vi "HostInteractiveOverlayedGraph.vi"(8 "stop_sign_queue":refnum<queue>, 11 "InputImg":i32[][](array[numeric])) -> (0 "Break":bool, 3 "Output_Coord":dbl[][](array[numeric]))   [LabVIEW 2024]
panel:
  in  "Revert":bool
  in  "stop":bool
  out "Image":i32[][](graph)
  out "Two Point Clicked?":bool
  in  "Ok":bool
  out "Point Clicked":i32
  in  "Reset":bool
  out "vidx":i32
  out "hidx":i32
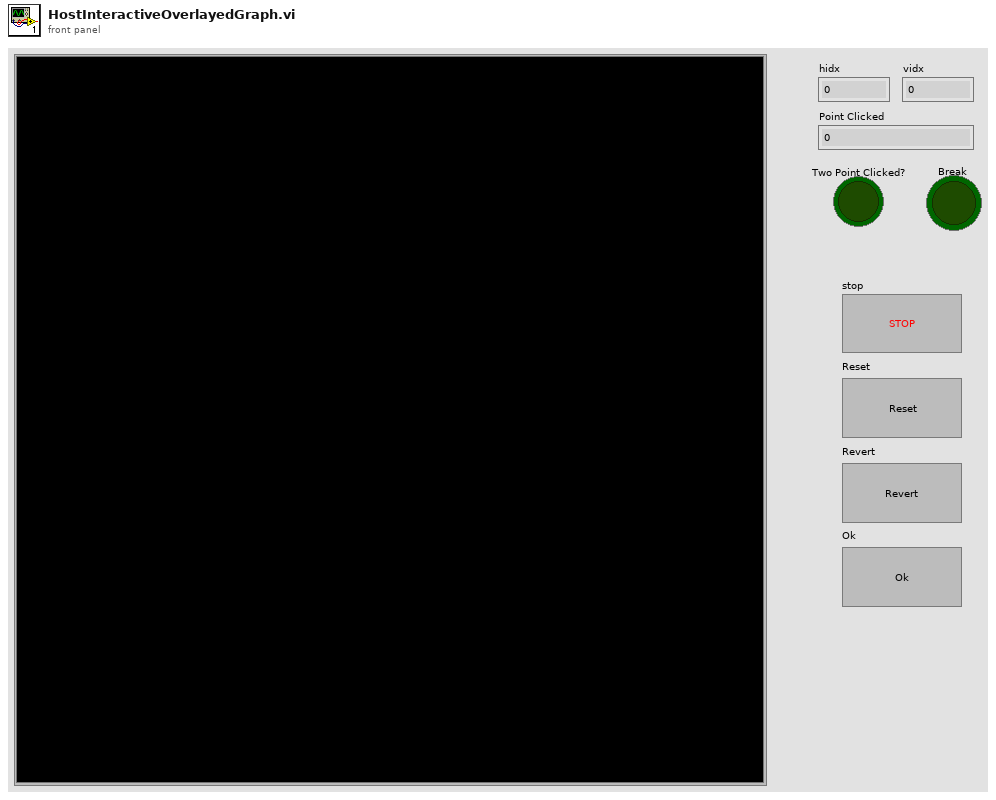
[diagram p1: front panel]
types:
  T1 = cluster{"Width":i16, "Style":enum32{"Solid", "Dash", "Dot", "DashDot", "DashDotDot"}}
  T2 = typedef "LVPoint32TypeDef.ctl" = cluster{"Horizontal":i32, "Vertical":i32}
  T3 = typedef "LVRectTypeDef.ctl" = cluster{"Left":i16, "Top":i16, "Right":i16, "Bottom":i16}
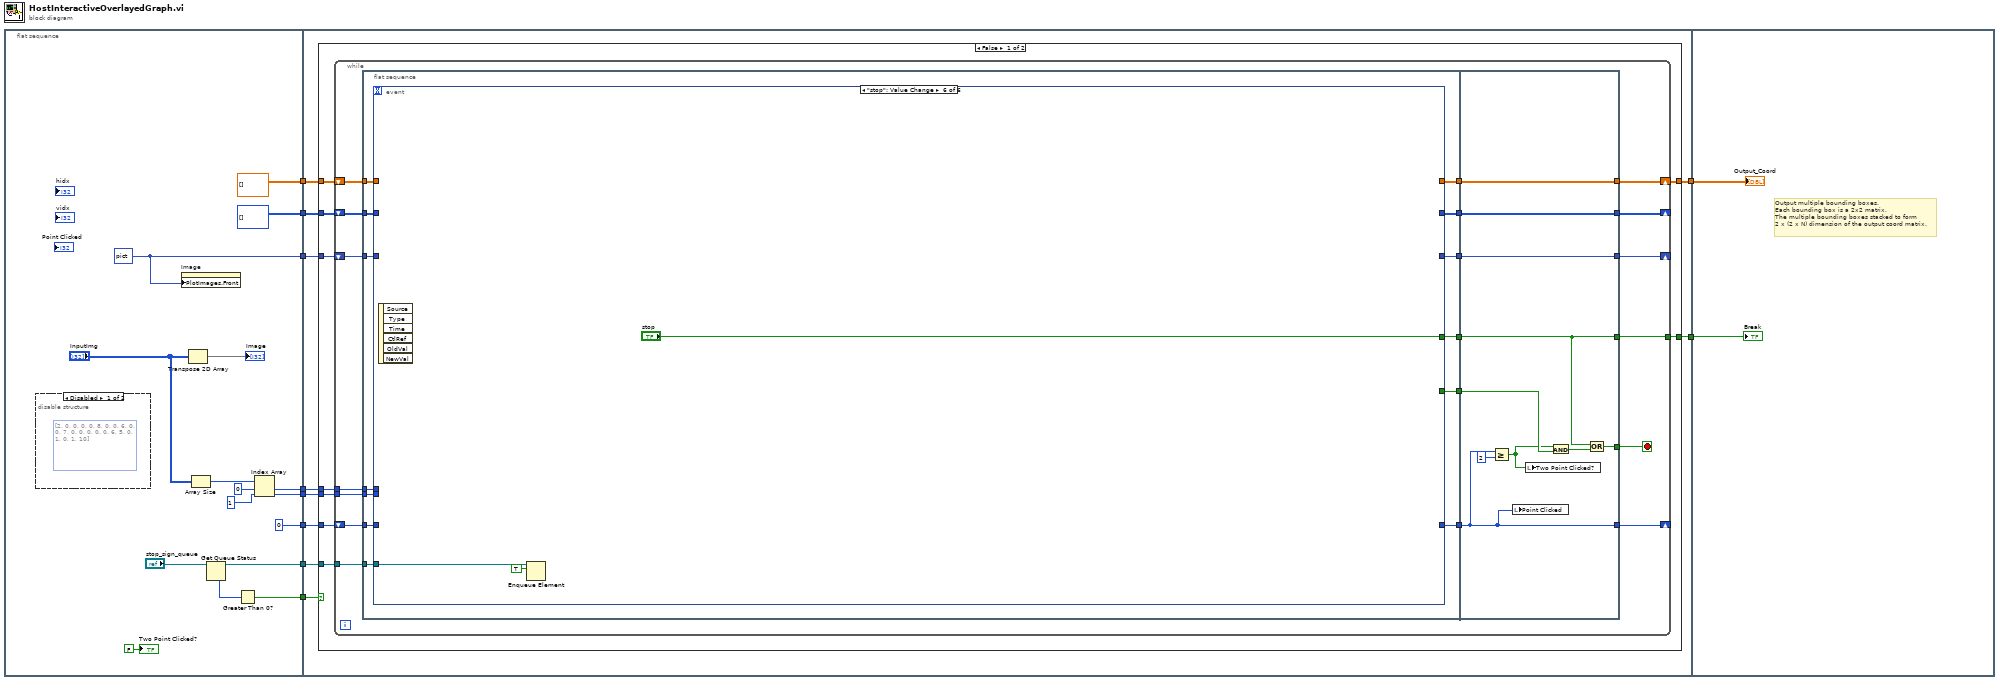
[diagram p0: block diagram]
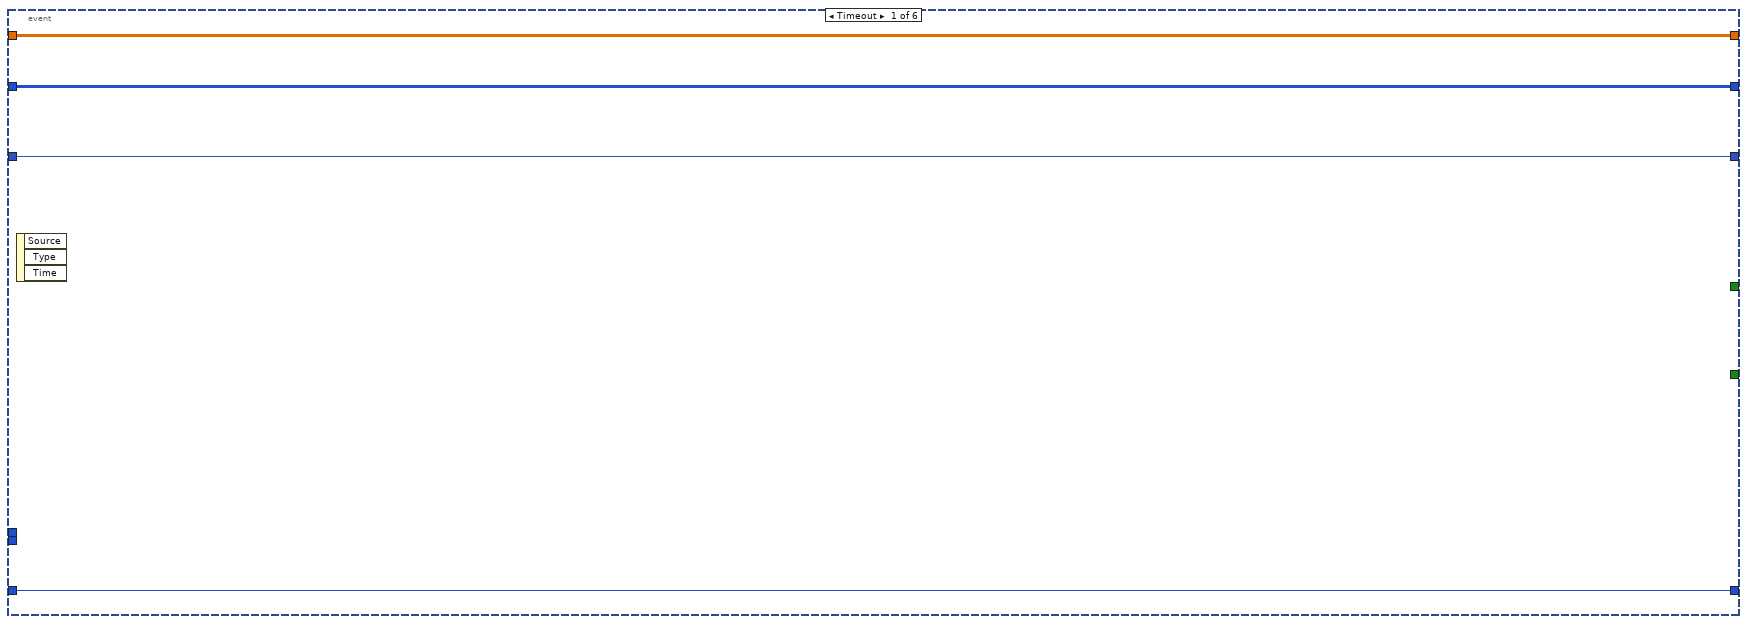
[diagram p3: hidden frame]
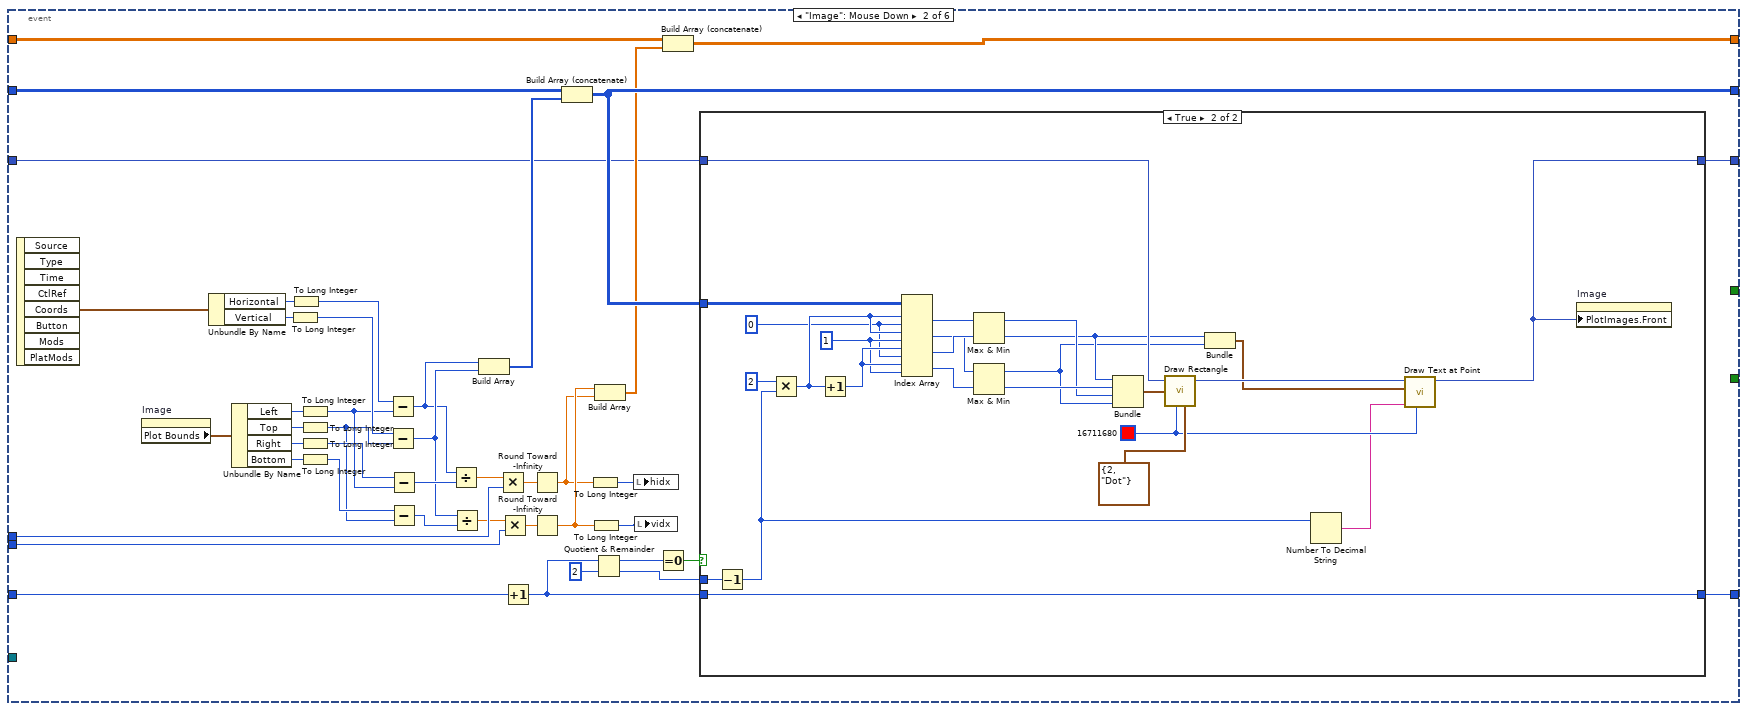
[diagram p4: hidden frame]
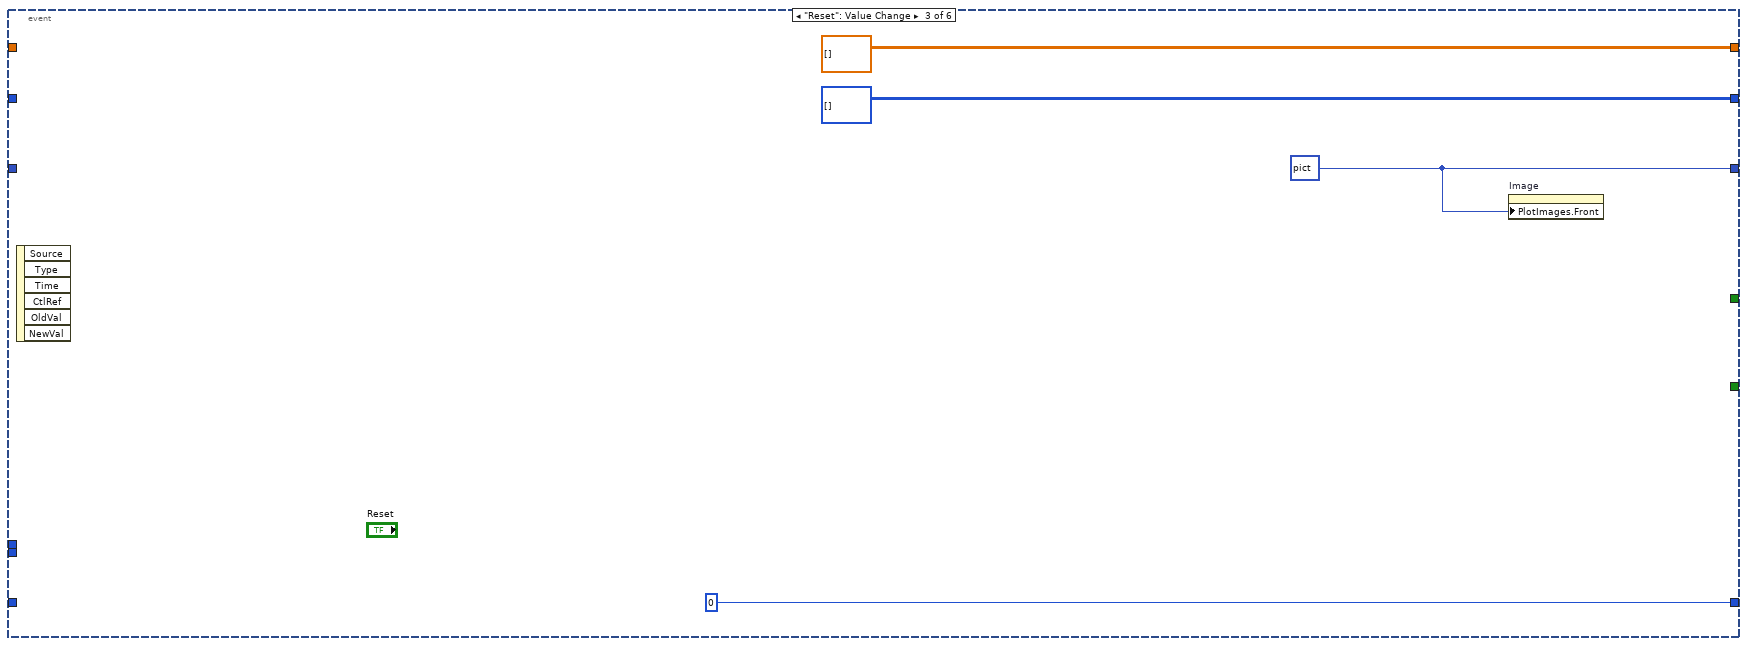
[diagram p6: hidden frame]
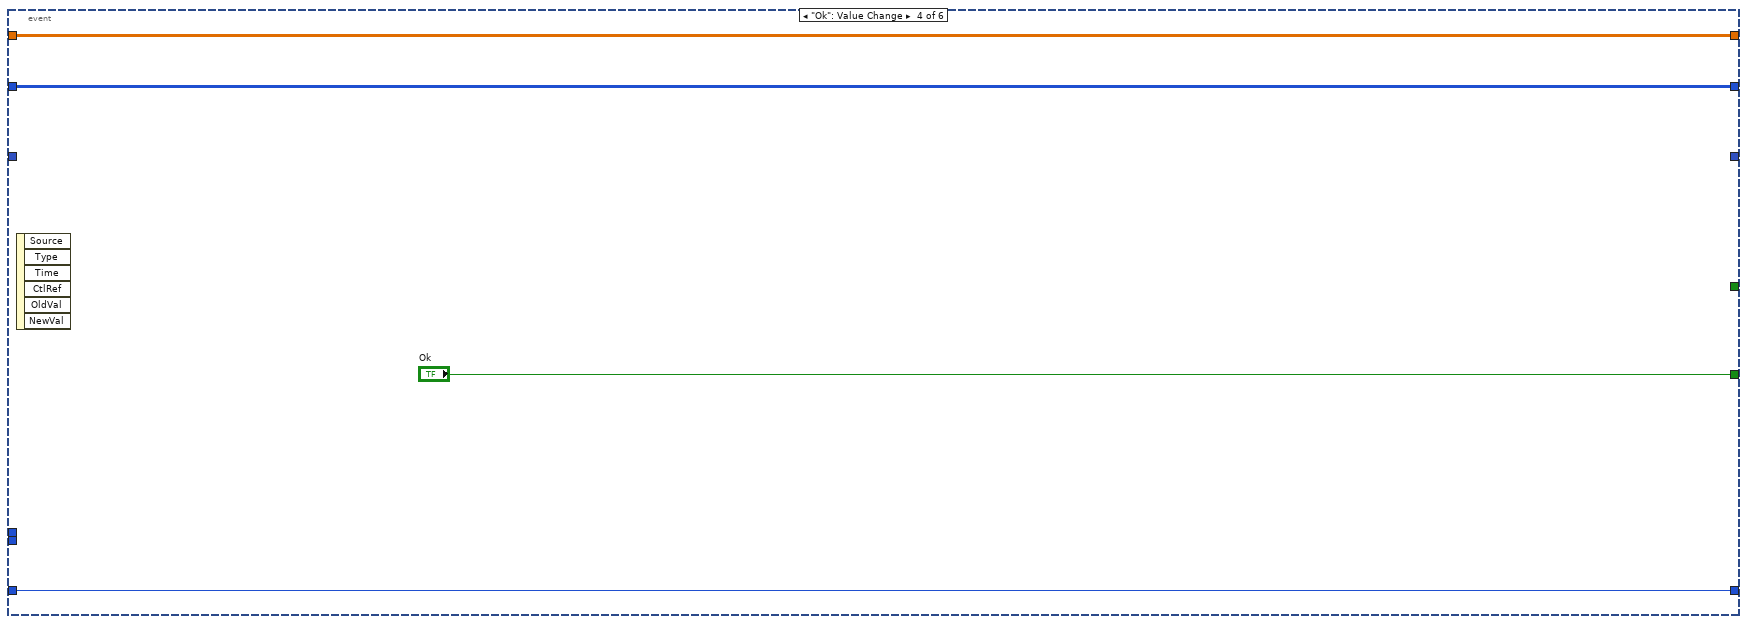
[diagram p7: hidden frame]
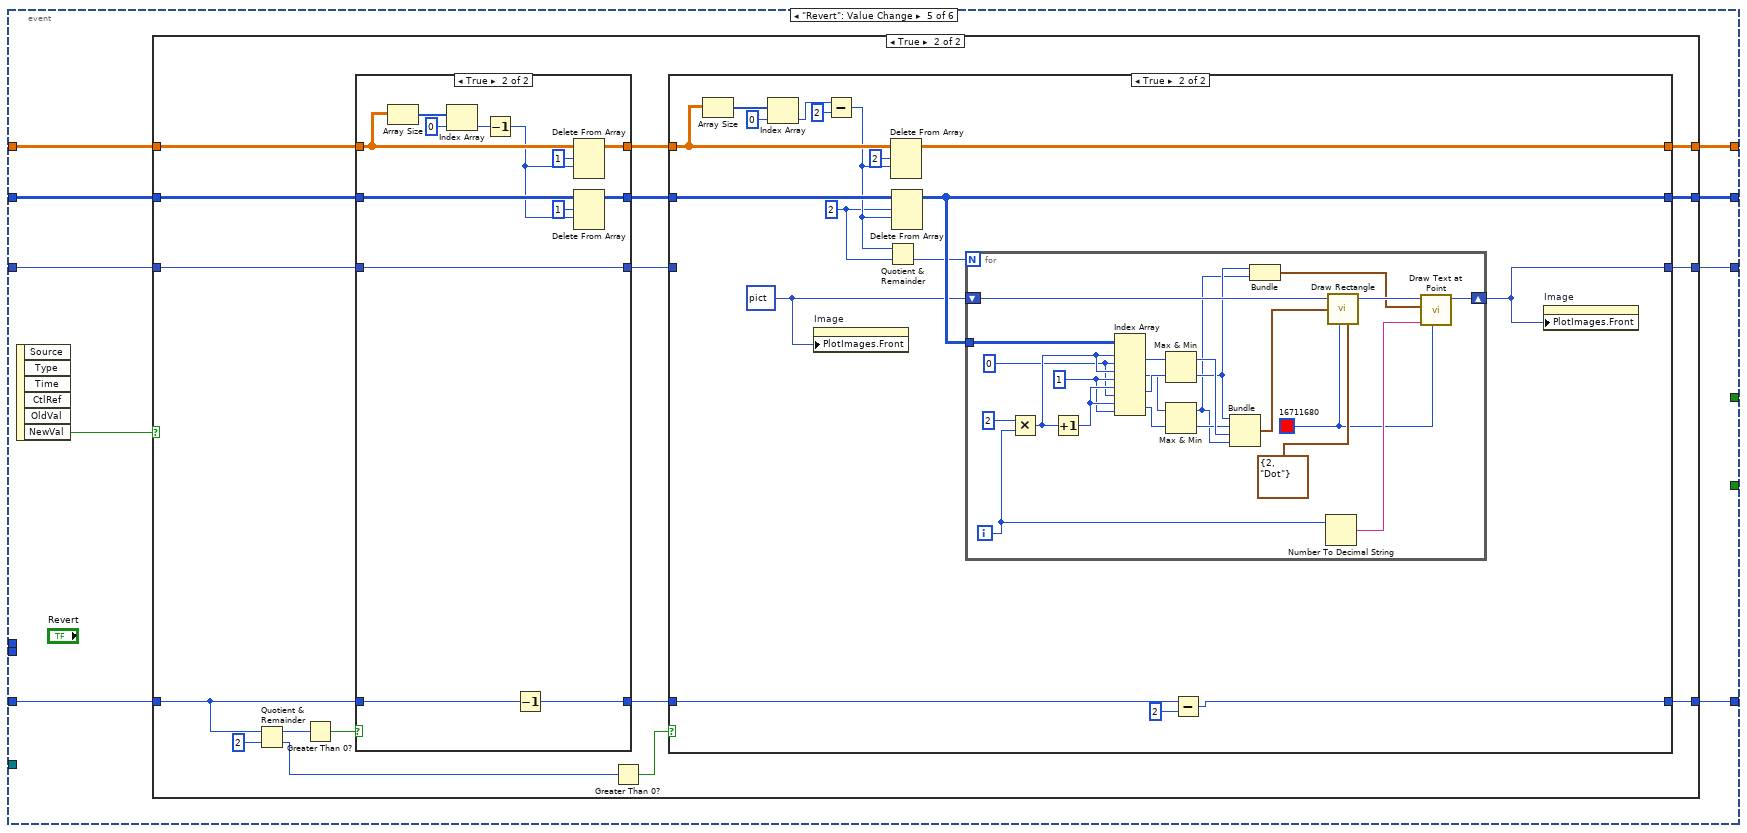
[diagram p8: hidden frame]
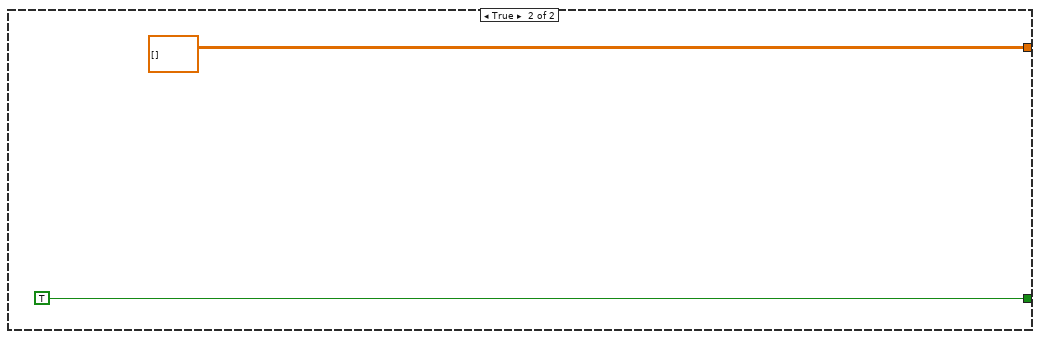
[diagram p12: hidden frame]
diagram:
  n1 = flat-sequence {
    tunnel: [w23] -> w10
    tunnel: [w22] -> w9
    tunnel: [0] -> w8
    tunnel: [dbl[][] []] -> w7
    tunnel: [w17] -> w4
    tunnel: [w16] -> w3
    tunnel: [i32[][] []] -> w2
    tunnel: [w14] -> w1
    tunnel: w10 -> [w36]
    tunnel: w9 -> [w35]
    tunnel: w8 -> [w34]
    tunnel: w7 -> [w33]
    tunnel: [w32] -> w6
    tunnel: [w31] -> w5
    tunnel: w4 -> [w30]
    tunnel: w3 -> [w29]
    tunnel: w2 -> [w28]
    tunnel: w1 -> [w27]
    tunnel: w6 -> [w267]
    tunnel: w5 -> [w266]
    frame #0 {
      w14 = picture data[5B] ("picture")
      n2 = disable-structure shown="Disabled" {
        frame Disabled {
          (unwired) i32[][] [[2, 0, 0, 0, 0, 8], [0, 0, 6, 0, 0, 7], [0, 0, 0, 0, 0, 6], [5, 0, 1, 0, 1, 10]]
        }
        frame Enabled {
        }
      }
      n3 = property on="Image" class="IntGraph (strict)"("PlotImages.Front"=w14) -> ()  [unwired: 2 in, 2 out]
      n4 = Transpose 2D Array(2D array="InputImg") -> (transposed array=→"Image":i32[][])
      n5 = Array Size(array="InputImg") -> (size(s)=w26:i32[])
      n6 = Get Queue Status(queue="stop_sign_queue") -> (queue out=w16:refnum<queue>, # elements in queue=w11:i32)  [unwired: 2 in, 6 out]
      n7 = Greater Than 0?(x=w11) -> (x > 0?=w17:bool)
      n8 = Index Array(array=w26, index #1=0 ("index"), index #2=1 ("index")) -> (element #1=w23:i32, element #2=w22:i32)
      "Two Point Clicked?" <- FALSE ("Two Point Clicked?")
    }
    frame #1 {
      n9 = case shown="False" w30 {
        tunnel: w36 -> [w45 _]
        tunnel: w35 -> [w44 _]
        tunnel: w34 -> [w43 _]
        tunnel: w33 -> [w42 _]
        tunnel: [w41 dbl[][] []] -> w32
        tunnel: [w40 TRUE ("stop")] -> w31
        tunnel: w29 -> [w39 _]
        tunnel: w28 -> [w38 _]
        tunnel: w27 -> [w37 _]
        frame False {
          n10 = while {
            tunnel: w45 -> [w64]
            tunnel: w44 -> [w63]
            shift-right: [w60] -> _
            shift-left: w43 -> [w62]
            shift-right: [w57] -> w41
            shift-left: w42 -> [w59]
            tunnel: [w53] -> w40
            tunnel: w39 -> [w52]
            shift-right: [w49] -> _
            shift-left: w38 -> [w51]
            shift-right: [w46] -> _
            shift-left: w37 -> [w48]
            stop <- w56 stop-if-true
            n11 = flat-sequence {
              tunnel: w64 -> [w77]
              tunnel: w63 -> [w76]
              tunnel: w62 -> [w75]
              tunnel: [w74] -> w61
              tunnel: w59 -> [w73]
              tunnel: [w72] -> w58
              tunnel: [w71] -> w55
              tunnel: [w70] -> w54
              tunnel: w52 -> [w69]
              tunnel: w51 -> [w68]
              tunnel: [w67] -> w50
              tunnel: w48 -> [w66]
              tunnel: [w65] -> w47
              tunnel: w61 -> [w254]
              tunnel: [w254] -> w60
              tunnel: w58 -> [w262]
              tunnel: [w262] -> w57
              tunnel: [w257] -> w56
              tunnel: w55 -> [w261]
              tunnel: w54 -> [w258]
              tunnel: [w258] -> w53
              tunnel: w50 -> [w256]
              tunnel: [w256] -> w49
              tunnel: w47 -> [w255]
              tunnel: [w255] -> w46
              frame #0 {
                n12 = event shown="[5] \"stop\": Value Change" {
                  selector: _ -> [_ _ _ _ _ _]
                  dyn-events: _ -> [_ _ _ _ _ _]
                  timeout: _ -> [_ _ _ _ _ _]
                  tunnel: w77 -> [_ w123 _ _ _ _]
                  tunnel: w76 -> [_ w122 _ _ _ _]
                  tunnel: w75 -> [w81 w119 _ w158 w168 _]
                  tunnel: [w81 w121 0 w158 w161 _] -> w74
                  tunnel: w73 -> [w80 w120 _ w159 w167 _]
                  tunnel: [w80 w118 dbl[][] [] w159 w164 _] -> w72
                  tunnel: [_ _ _ "Ok" _ _] -> w71
                  tunnel: [_ _ _ _ _ "stop"] -> w70
                  tunnel: w69 -> [_ _ _ _ _ w252]
                  tunnel: w68 -> [w79 w117 _ w156 w166 _]
                  tunnel: [w79 w116 i32[][] [] w156 w163 _] -> w67
                  tunnel: w66 -> [w78 w85 _ _ w165 _]
                  tunnel: [w78 w84 w152 _ w162 _] -> w65
                  event Timeout {
                    n13 = event-data() -> ()  [unwired: 1 in, 3 out]
                  }
                  event "Image": Mouse Down {
                    n14 = event-data() -> ("Coords"=w124:T2)  [unwired: 1 in, 7 out]
                    n15 = property on="Image" class="IntGraph (strict)"() -> ("Plot Bounds"=w96:T3)  [unwired: 2 in, 2 out]
                    n16 = Unbundle By Name(w124) -> ("Horizontal"=w115:i32, "Vertical"=w113:i32)
                    n17 = Unbundle By Name(w96) -> ("Left"=w111:i16, "Top"=w110:i16, "Right"=w109:i16, "Bottom"=w108:i16)
                    n18 = To Long Integer(number=w113) -> (32bit integer=w112:i32)
                    n19 = To Long Integer(number=w115) -> (32bit integer=w114:i32)
                    n20 = To Long Integer(number=w111) -> (32bit integer=w107:i32)
                    n21 = To Long Integer(number=w110) -> (32bit integer=w100:i32)
                    n22 = To Long Integer(number=w109) -> (32bit integer=w105:i32)
                    n23 = To Long Integer(number=w108) -> (32bit integer=w106:i32)
                    n24 = Subtract(x=w114, y=w107) -> (x-y=w86:i32)
                    n25 = Subtract(x=w112, y=w100) -> (x-y=w92:i32)
                    n26 = Subtract(x=w105, y=w107) -> (x-y=w104:i32)
                    n27 = Subtract(x=w106, y=w100) -> (x-y=w101:i32)
                    n28 = Divide(x=w86, y=w104) -> (x/y=w103:dbl)
                    n29 = Divide(x=w92, y=w101) -> (x/y=w102:dbl)
                    n30 = Build Array(w86, w92) -> (w93:i32[])
                    n31 = Multiply(x=w103, y=w123) -> (x*y=w99:dbl)
                    n32 = Multiply(x=w102, y=w122) -> (x*y=w98:dbl)
                    n33 = Increment(x=w119) -> (x+1=w88:i32)
                    n34 = Round Toward -Infinity(1:w99) -> (0:w94:dbl)
                    n35 = Round Toward -Infinity(1:w98) -> (0:w95:dbl)
                    n36 = Build Array (concatenate)(w117, w93) -> (w116:i32[][])
                    n37 = To Long Integer(number=w94) -> (32bit integer=w83:i32)
                    n38 = To Long Integer(number=w95) -> (32bit integer=w82:i32)
                    n39 = Quotient & Remainder(x=w88, y=2) -> (x-y*floor(x/y)=w90:i32, floor(x/y)=w87:i32)
                    n40 = Build Array(w95, w94) -> (w97:dbl[])
                    n41 = local write "hidx"(w83) -> ()
                    n42 = local write "vidx"(w82) -> ()
                    n43 = Equal To 0?(x=w90) -> (x = 0?=w89:bool)
                    n44 = Build Array (concatenate)(w120, w97) -> (w118:dbl[][])
                    n45 = case shown="True" w89 {
                      tunnel: w116 -> [_ w151]
                      tunnel: w88 -> [w126 w149]
                      tunnel: [w126 w149] -> w121
                      tunnel: w87 -> [_ w145]
                      tunnel: w85 -> [w125 w135]
                      tunnel: [w125 w133] -> w84
                      frame False {
                      }
                      frame True {
                        w144 = 1 ("disabled index (col)")
                        w136 = 0 ("disabled index (col)")
                        w132 = u32 16711680 ("color(black)")
                        n46 = Decrement(x=w145) -> (x-1=w131:i32)
                        n47 = Multiply(x=2 ("y"), y=w131) -> (x*y=w147:i32)
                        n48 = Increment(x=w147) -> (x+1=w146:i32)
                        n49 = Index Array(array=w151, index (row) #1=w147, index (col) #1=w136, index (row) #2=w147, index (col) #2=w144, index (row) #3=w146, index (col) #3=w136, index (row) #4=w146, index (col) #4=w144) -> (element #1=w143:i32, element #2=w139:i32, element #3=w140:i32, element #4=w142:i32)
                        n50 = Max & Min(x=w143, y=w140) -> (max(x,y)=w137:i32, min(x,y)=w129:i32)
                        n51 = Max & Min(x=w139, y=w142) -> (max(x,y)=w128:i32, min(x,y)=w138:i32)
                        n52 = Bundle(w129, w138, w137, w128) -> (w150:cluster{i32, i32, i32, i32})  [unwired: 1 in]
                        n53 = call <vilib>:"Draw Rectangle.vi"("picture"=w135, "rect"=w150, "color(black)"=w132, "pen"=T1 {"Width"=2, "Style"=enum."Dot"}) -> ("new picture"=w134:picture)  [unwired: 5 in]
                        n54 = Bundle(w129, w128) -> (w127:cluster{i32, i32})  [unwired: 1 in]
                        n55 = Number To Decimal String(number=w131) -> (decimal integer string=w130:string)  [unwired: 1 in]
                        n56 = call <vilib>:"Draw Text at Point.vi"("text color(black)"=w132, "text"=w130, "origin"=w127, "picture"=w134) -> ("new picture"=w133:picture)  [unwired: 6 in, 1 out]
                        n57 = property on="Image" class="IntGraph (strict)"("PlotImages.Front"=w133) -> ()  [unwired: 2 in, 2 out]
                      }
                    }
                  }
                  event "Reset": Value Change {
                    w152 = picture data[5B] ("picture")
                    n58 = event-data() -> ()  [unwired: 1 in, 6 out]
                    n59 = property on="Image" class="IntGraph (strict)"("PlotImages.Front"=w152) -> ()  [unwired: 2 in, 2 out]
                  }
                  event "Ok": Value Change {
                    n60 = event-data() -> ()  [unwired: 1 in, 6 out]
                  }
                  event "Revert": Value Change {
                    n61 = event-data() -> ("NewVal"=w160:bool)  [unwired: 1 in, 5 out]
                    n62 = case shown="True" w160 {
                      tunnel: w168 -> [w169 w186]
                      tunnel: w167 -> [w172 w185]
                      tunnel: w166 -> [w171 w184]
                      tunnel: w165 -> [w170 w183]
                      tunnel: [w172 w176] -> w164
                      tunnel: [w171 w175] -> w163
                      tunnel: [w170 w174] -> w162
                      tunnel: [w169 w173] -> w161
                      frame False {
                      }
                      frame True {
                        n63 = Quotient & Remainder(x=w186, y=2) -> (x-y*floor(x/y)=w188:i32, floor(x/y)=w182:i32)
                        n64 = Greater Than 0?(x=w188) -> (x > 0?=w187:bool)
                        n65 = case shown="True" w187 {
                          tunnel: w186 -> [w237 w250]
                          tunnel: [w237 w249] -> w180
                          tunnel: w185 -> [w236 w247]
                          tunnel: w184 -> [w235 w248]
                          tunnel: w183 -> [w234 w240]
                          tunnel: [w236 w242] -> w179
                          tunnel: [w235 w241] -> w178
                          tunnel: [w234 w240] -> w177
                          frame False {
                          }
                          frame True {
                            n66 = Array Size(array=w247) -> (size(s)=w246:i32[])
                            n67 = Index Array(array=w246, index=0) -> (element=w239:i32)
                            n68 = Decrement(x=w239) -> (x-1=w238:i32)
                            n69 = Decrement(x=w250) -> (x-1=w249:i32)
                            n70 = Delete From Array(array=w247, length=1, index (row)=w238) -> (array with subset deleted=w242:dbl[][])  [unwired: 1 in, 1 out]
                            n71 = Delete From Array(array=w248, length=1, index (row)=w238) -> (array with subset deleted=w241:i32[][])  [unwired: 1 in, 1 out]
                          }
                        }
                        n72 = Greater Than 0?(x=w182) -> (x > 0?=w181:bool)
                        n73 = case shown="True" w181 {
                          tunnel: w180 -> [w193 w210]
                          tunnel: [w193 w208] -> w173
                          tunnel: w179 -> [w190 w203]
                          tunnel: w178 -> [w191 w201]
                          tunnel: w177 -> [w192 _]
                          tunnel: [w192 w198] -> w174
                          tunnel: [w191 w199] -> w175
                          tunnel: [w190 w200] -> w176
                          frame False {
                          }
                          frame True {
                            w195 = 2 ("length")
                            w197 = picture data[5B] ("picture")
                            n74 = Array Size(array=w203) -> (size(s)=w206:i32[])
                            n75 = Index Array(array=w206, index=0) -> (element=w205:i32)
                            n76 = property on="Image" class="IntGraph (strict)"("PlotImages.Front"=w197) -> ()  [unwired: 2 in, 2 out]
                            n77 = Subtract(x=w205, y=2) -> (x-y=w196:i32)
                            n78 = Quotient & Remainder(x=w196, y=w195) -> (floor(x/y)=w194:i32)  [unwired: 1 out]
                            n79 = Delete From Array(array=w203, length=2, index (row)=w196) -> (array with subset deleted=w200:dbl[][])  [unwired: 1 in, 1 out]
                            n80 = Delete From Array(array=w201, length=w195, index (row)=w196) -> (array with subset deleted=w199:i32[][])  [unwired: 1 in, 1 out]
                            n81 = for {
                              N: w194 -> [_]
                              tunnel: w199 -> [w223]
                              shift-right: [w216] -> w198
                              shift-left: w197 -> [w222]
                              i -> [w215]
                              w212 = u32 16711680 ("color(black)")
                              w230 = 1 ("disabled index (col)")
                              w224 = 0 ("disabled index (col)")
                              n82 = Multiply(x=2 ("y"), y=w215) -> (x*y=w232:i32)
                              n83 = Increment(x=w232) -> (x+1=w231:i32)
                              n84 = Index Array(array=w223, index (row) #1=w232, index (col) #1=w224, index (row) #2=w232, index (col) #2=w230, index (row) #3=w231, index (col) #3=w224, index (row) #4=w231, index (col) #4=w230) -> (element #1=w229:i32, element #2=w226:i32, element #3=w227:i32, element #4=w228:i32)
                              n85 = Max & Min(x=w229, y=w227) -> (max(x,y)=w225:i32, min(x,y)=w219:i32)
                              n86 = Max & Min(x=w226, y=w228) -> (max(x,y)=w211:i32, min(x,y)=w218:i32)
                              n87 = Bundle(w219, w218, w225, w211) -> (w221:cluster{i32, i32, i32, i32})  [unwired: 1 in]
                              n88 = Bundle(w219, w211) -> (w213:cluster{i32, i32})  [unwired: 1 in]
                              n89 = Number To Decimal String(number=w215) -> (decimal integer string=w214:string)  [unwired: 1 in]
                              n90 = call <vilib>:"Draw Rectangle.vi"("picture"=w222, "rect"=w221, "color(black)"=w212, "pen"=T1 {"Width"=2, "Style"=enum."Dot"}) -> ("new picture"=w217:picture)  [unwired: 5 in]
                              n91 = call <vilib>:"Draw Text at Point.vi"("text color(black)"=w212, "text"=w214, "origin"=w213, "picture"=w217) -> ("new picture"=w216:picture)  [unwired: 6 in, 1 out]
                            }
                            n92 = Subtract(x=w210, y=2) -> (x-y=w208:i32)
                            n93 = property on="Image" class="IntGraph (strict)"("PlotImages.Front"=w198) -> ()  [unwired: 2 in, 2 out]
                          }
                        }
                      }
                    }
                  }
                  event "stop": Value Change {
                    n94 = event-data() -> ()  [unwired: 1 in, 6 out]
                    n95 = Enqueue Element(queue=w252, element=TRUE) -> ()  [unwired: 2 in, 3 out]
                  }
                }
              }
              frame #1 {
                n96 = Greater Or Equal?(x=w254, y=2) -> (x >= y?=w260:bool)
                n97 = local write "Point Clicked"(w254) -> ()
                n98 = local write "Two Point Clicked?"(w260) -> ()
                n99 = And(x=w260, y=w261) -> (x .and. y?=w259:bool)
                n100 = Or(x=w258, y=w259) -> (x .or. y?=w257:bool)
              }
            }
          }
        }
        frame True {
        }
      }
    }
    frame #2 {
      # "Output multiple bounding boxes.\nEach bounding box is a 2x2 matrix. \nThe multiple bounding boxes stacked to form \n2 x (2 x N) dimension of the output coord matrix."
      "Output_Coord" <- w267
      "Break" <- w266
    }
  }
